vi "search_string_value.vi"(8 "索引项":string, 11 "数组":cluster{"String":string, "Value":dbl}[](array[cluster])) -> (2 "索引值":dbl)   [LabVIEW 2016, in "MotionControl.lvlib" / "StepMotor.lvclass"]
uses:
  <userlib>/MotionControl/StepMotor/StepMotor.lvclass
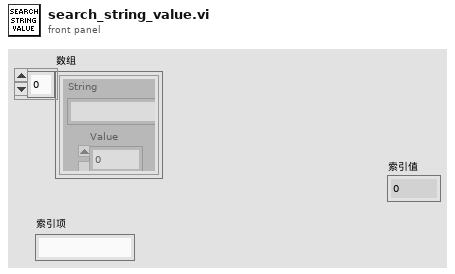
[diagram p1: front panel]
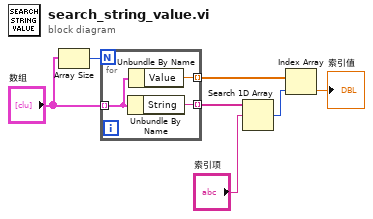
[diagram p0: block diagram]
diagram:
  n1 = Array Size(array="数组") -> (size(s)=w1:i32)
  n2 = for {
    N: w1 -> [_]
    tunnel: [w10] -> w7 mode=indexing
    tunnel: [w9] -> w5 mode=indexing
    tunnel: "数组" -> [w8] mode=indexing
    n3 = Unbundle By Name(w8) -> ("String"=w10:string)
    n4 = Unbundle By Name(w8) -> ("Value"=w9:dbl)
  }
  n5 = Search 1D Array(1D array=w7, element="索引项") -> (index of element=w4:i32)  [unwired: 1 in]
  n6 = Index Array(array=w5, index=w4) -> (element=→"索引值":dbl)
